vi "Configure Temperature Offset.vi"(8 "error in (no error)":errorcluster, 10 "offset, °C":dbl, 11 "HECR in":refnum<class "PL SMC HECR.lvclass">) -> (0 "error out":errorcluster, 3 "HECR out":refnum<class "PL SMC HECR.lvclass">)   [LabVIEW 2015, in "PL SMC HECR.lvclass"]
doc: "Configures temperature offset."
uses:
  PL SMC HECR.lvclass
  <vilib>/plasmapper/PL Modbus Client/PL Modbus Client.lvclass
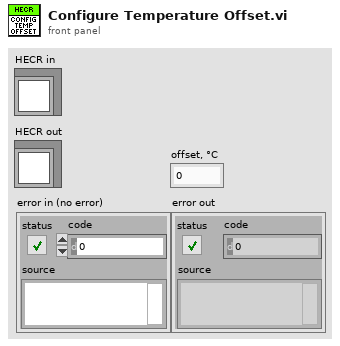
[diagram p1: front panel]
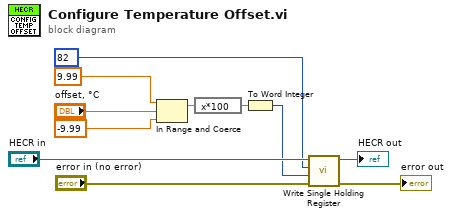
[diagram p0: block diagram]
diagram:
  n1 = In Range and Coerce(upper limit=9.99 ("Ttarget, °C"), x="offset, °C", lower limit=-9.99 ("Ttarget, °C")) -> (coerced(x)=w6:dbl)  [unwired: 1 out]
  n2 = expression code="x*100"(w6) -> (w2:dbl)
  n3 = To Word Integer(number=w2) -> (16bit integer=w1:i16)
  n4 = call <vilib>:"Write Single Holding Register.vi"("error in (no error)"="error in (no error)", "value"=w1, "address"=u16 82, "MODBUS in"="HECR in") -> ("error out"=→"error out":errorcluster, "MODBUS out"=→"HECR out":refnum<class "PL SMC HECR.lvclass">)  [unwired: 6 in]
